vi "AxisSteps.vi"() -> ()   [LabVIEW 2011]
panel:
  in  "X Mirror_Steps":dbl
  in  "Y_Mirror_Steps":dbl
  in  "Stack_Scanner_Steps":dbl
  in  "Slow_Scanner_Steps":dbl
  in  "Fast_Scanner_Steps":dbl
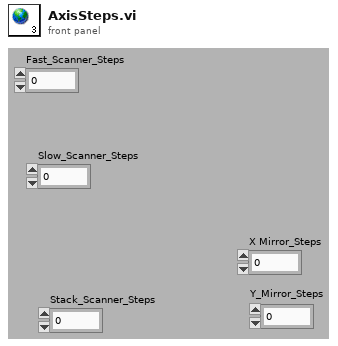
[diagram p1: front panel]
diagram:
